vi "_Highlight CSM Scripts(StringControl).vi"(11 "String Ctrl":refnum<vi>) -> ()   [LabVIEW 2017]
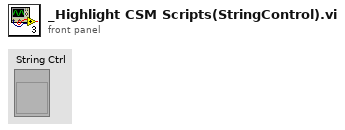
[diagram p1: front panel]
types:
  T1 = cluster{"Text.Selection:Start":u32, "Text.Selection:End":u32, "cb":u32, "underline":bool, "Italic":bool, "Bold":bool}[]
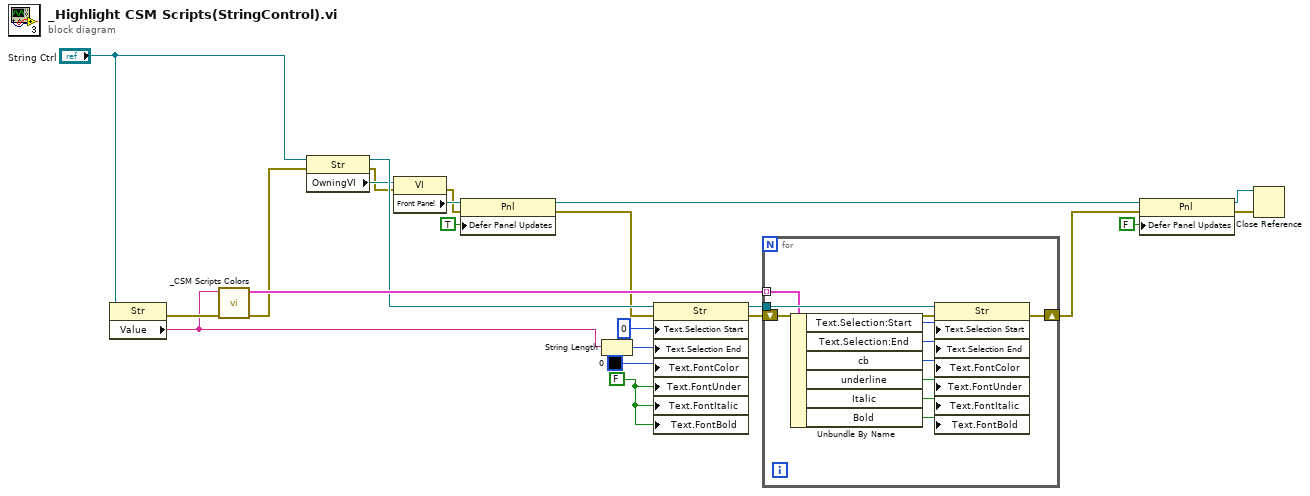
[diagram p0: block diagram]
diagram:
  w15 = FALSE ("Text.Font:Underline")
  n1 = property class="Str"(reference="String Ctrl") -> (error out=w23:errorcluster, "Value"=w17:string)  [unwired: 1 in, 1 out]
  n2 = call "_CSM Scripts Colors.vi"("Error in"=w23, "Value"=w17) -> ("Error out"=w10:errorcluster, "Array"=w22:T1)  [unwired: 8 in]
  n3 = property class="Str"(reference="String Ctrl", error in=w10) -> (reference out=w13:refnum<vi>, error out=w7:errorcluster, "OwningVI"=w12:refnum<vi>)
  n4 = property class="VI"(reference=w12, error in=w7) -> (error out=w8:errorcluster, "Front Panel"=w11:refnum<vi>)  [unwired: 1 out]
  n5 = property class="Pnl"(reference=w11, error in=w8, "Defer Panel Updates"=TRUE) -> (reference out=w3:refnum<vi>, error out=w6:errorcluster)
  n6 = String Length(string=w17) -> (length=w18:i32)
  n7 = property class="Str"(reference=w13, error in=w6, "Text.Selection Start"=u32 0 ("Text.Selection:Start"), "Text.Selection End"=w18, "Text.FontColor"=u32 0, "Text.FontUnder"=w15, "Text.FontItalic"=w15, "Text.FontBold"=w15) -> (reference out=w20:refnum<vi>, error out=w21:errorcluster)
  n8 = for {
    tunnel: w20 -> [w33]
    tunnel: w22 -> [w31] mode=indexing
    shift-right: [w24] -> w4
    shift-left: w21 -> [w32]
    n9 = Unbundle By Name(w31) -> ("Text.Selection:Start"=w30:u32, "Text.Selection:End"=w29:u32, "cb"=w28:u32, "underline"=w27:bool, "Italic"=w26:bool, "Bold"=w25:bool)
    n10 = property class="Str"(reference=w33, error in=w32, "Text.Selection Start"=w30, "Text.Selection End"=w29, "Text.FontColor"=w28, "Text.FontUnder"=w27, "Text.FontItalic"=w26, "Text.FontBold"=w25) -> (error out=w24:errorcluster)  [unwired: 1 out]
  }
  n11 = property class="Pnl"(reference=w3, error in=w4, "Defer Panel Updates"=FALSE) -> (reference out=w1:refnum<vi>, error out=w2:errorcluster)
  n12 = Close Reference(reference=w1, error in (no error)=w2) -> ()  [unwired: 1 out]
